vi "Multitone Eval.vi"(8 "error in (no error)":errorcluster, 9 "phase":dbl[](array[numeric]), 10 "frequency":dbl[](array[numeric]), 11 "amplitude":dbl[](array[numeric])) -> (0 "error out":errorcluster, 3 "String":string)   [LabVIEW 2016, in "Lockin.DAQ.lvclass"]
uses:
  Lockin.DAQ.lvclass
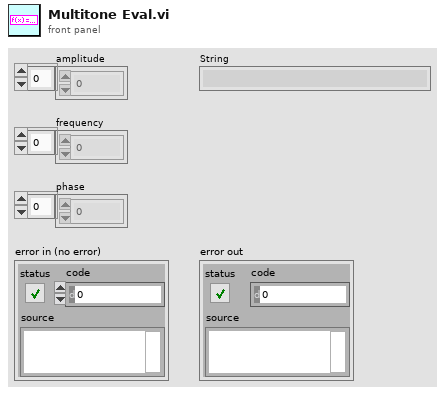
[diagram p1: front panel]
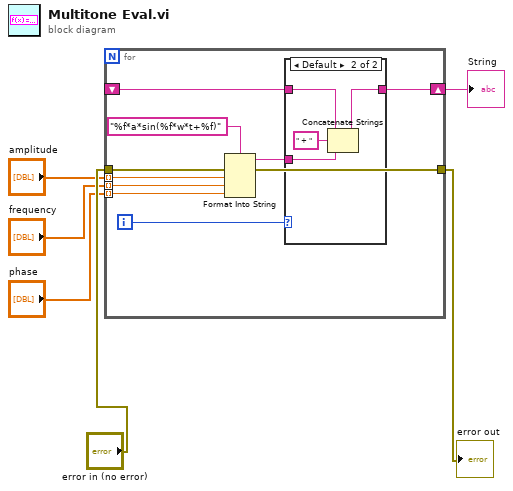
[diagram p0: block diagram]
diagram:
  n1 = for {
    tunnel: "phase" -> [w15] mode=indexing
    tunnel: "amplitude" -> [w14] mode=indexing
    tunnel: "frequency" -> [w13] mode=indexing
    shift-right: [w11] -> w1
    shift-left: _ -> [w10]
    tunnel: "error in (no error)" -> [w8]
    tunnel: [w7] -> w6
    i -> [w9]
    n2 = Format Into String(format string="%f*a*sin(%f*w*t+%f)" ("formula"), error in=w8, w14, w13, w15) -> (resulting string=w12:string, error out=w7:errorcluster)  [unwired: 1 in]
    n3 = case shown="Default" w9 {
      tunnel: w12 -> [w17 w21]
      tunnel: [w17 w18] -> w11
      tunnel: w10 -> [_ w20]
      frame 0 {
      }
      frame Default {
        n4 = Concatenate Strings(w20, " + " ("string"), w21) -> (w18:string)
      }
    }
  }
  "error out" <- w6
  "String" <- w1
